vi "Write Read Delay.vi"(0 "Visa Ref":refnum<visa-resource-name>, 2 "Conversion (steps/ns)":dbl format="%#_13g", 7 "Delay (ns)":dbl, 11 "Gate Delay Actions":T1) -> (4 "Visa Ref Dup":refnum<visa-resource-name>, 8 "Delay Out (ns)":dbl)   [LabVIEW 2016]
uses:
  Gate Delay Type Defs/Gate Delay Actions.ctl
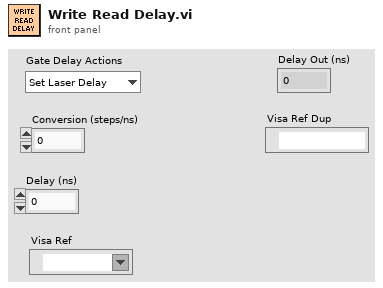
[diagram p1: front panel]
types:
  T1 = typedef "Gate Delay Actions.ctl" = enum16{"Set Laser Delay", "Set Window Delay", "Set Window Width", "Get Delays", "Set Default Delays", "Restore Defaults", "Quit"}
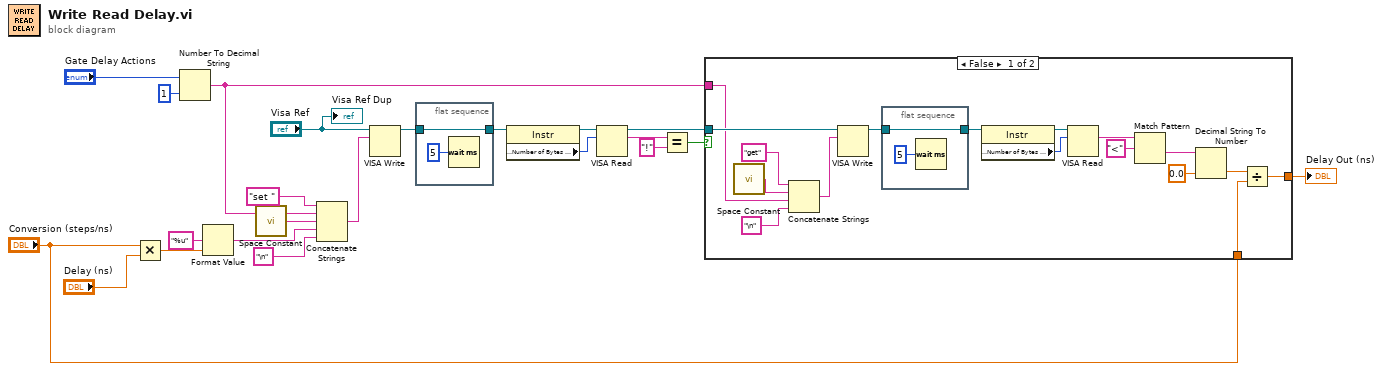
[diagram p0: block diagram]
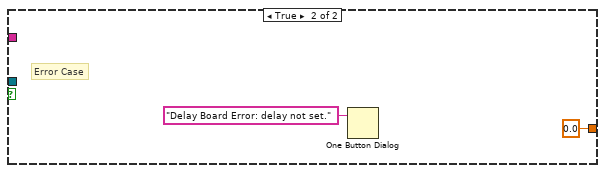
[diagram p2: hidden frame]
diagram:
  n1 = Multiply(x="Conversion (steps/ns)", y="Delay (ns)") -> (x*y=w10:dbl)
  n2 = Number To Decimal String(number="Gate Delay Actions", width (-)=i16 1) -> (decimal integer string=w3:string)
  n3 = Format Value(format string="%u", value (0)=w10) -> (output string=w9:string)  [unwired: 1 in]
  n4 = call <vilib>:"Space Constant.vi"() -> ("String"=w22:string)
  n5 = Concatenate Strings("set ", w3, w22, w9, "\n") -> (w14:string)
  n6 = VISA Write(VISA resource name="Visa Ref", write buffer=w14) -> (VISA resource name out=w17:refnum<visa-resource-name>)  [unwired: 1 in, 2 out]
  n7 = flat-sequence {
    tunnel: [w24] -> w18
    tunnel: w17 -> [w24]
    frame #0 {
      n8 = Wait (ms)(milliseconds to wait=u32 5) -> ()  [unwired: 1 out]
    }
  }
  n9 = property class="Instr"(reference=w18) -> (reference out=w16:refnum<visa-resource-name>, "Serial Settings:Number of Bytes at Serial Port"=w15:u32)  [unwired: 1 in, 1 out]
  n10 = VISA Read(VISA resource name=w16, byte count=w15) -> (VISA resource name out=w4:refnum<visa-resource-name>, read buffer=w20:string)  [unwired: 1 in, 2 out]
  n11 = Equal?(x=w20, y="!") -> (x = y?=w5:bool)
  n12 = case shown="False" w5 {
    tunnel: w4 -> [w35 _]
    tunnel: w3 -> [w31 _]
    tunnel: "Conversion (steps/ns)" -> [w27 _]
    tunnel: [w26 0.0] -> w1
    frame False {
      n13 = call <vilib>:"Space Constant.vi"() -> ("String"=w33:string)
      n14 = Concatenate Strings("get" ("string"), w33, w31, "\n") -> (w30:string)
      n15 = VISA Write(VISA resource name=w35, write buffer=w30) -> (VISA resource name out=w41:refnum<visa-resource-name>)  [unwired: 1 in, 2 out]
      n16 = flat-sequence {
        tunnel: [w43] -> w40
        tunnel: w41 -> [w43]
        frame #0 {
          n17 = Wait (ms)(milliseconds to wait=u32 5) -> ()  [unwired: 1 out]
        }
      }
      n18 = property class="Instr"(reference=w40) -> (reference out=w25:refnum<visa-resource-name>, "Serial Settings:Number of Bytes at Serial Port"=w39:u32)  [unwired: 1 in, 1 out]
      n19 = VISA Read(VISA resource name=w25, byte count=w39) -> (read buffer=w38:string)  [unwired: 1 in, 3 out]
      n20 = Match Pattern(string=w38, regular expression="<") -> (after substring=w36:string)  [unwired: 1 in, 3 out]
      n21 = Decimal String To Number(string=w36, default (0L)=0.0) -> (number=w28:dbl)  [unwired: 1 in, 1 out]
      n22 = Divide(x=w28, y=w27) -> (x/y=w26:dbl)
    }
    frame True {
      # "Error Case"
      n23 = One Button Dialog(message="Delay Board Error: delay not set.") -> ()  [unwired: 1 in, 1 out]
    }
  }
  "Delay Out (ns)" <- w1
  "Visa Ref Dup" <- "Visa Ref"
